vi "InsertMTtemp2DB.vi"(8 "error in (no error)":errorcluster, 9 "Entity":string="QAMT03", 11 "file (use dialog)":path=path "C:/temp/RunTemp/TesterTempByNow.txt") -> (0 "error out":errorcluster)   [LabVIEW 2012]
uses:
  <vilib>/Utility/file.llb/Read From Spreadsheet File (string).vi
  <vilib>/addons/database/Connection.llb/DB Tools Open Connec (Path).vi
  <vilib>/addons/database/Connection.llb/Conn Execute.vi
  <vilib>/addons/database/Recordset.llb/Rec Fetch Integer Data (R).vi
  <vilib>/addons/database/Recordset.llb/Rec Destroy - Connection.vi
  <vilib>/addons/database/NI_Database_API.lvlib
panel:
  in  "Cluster":T1
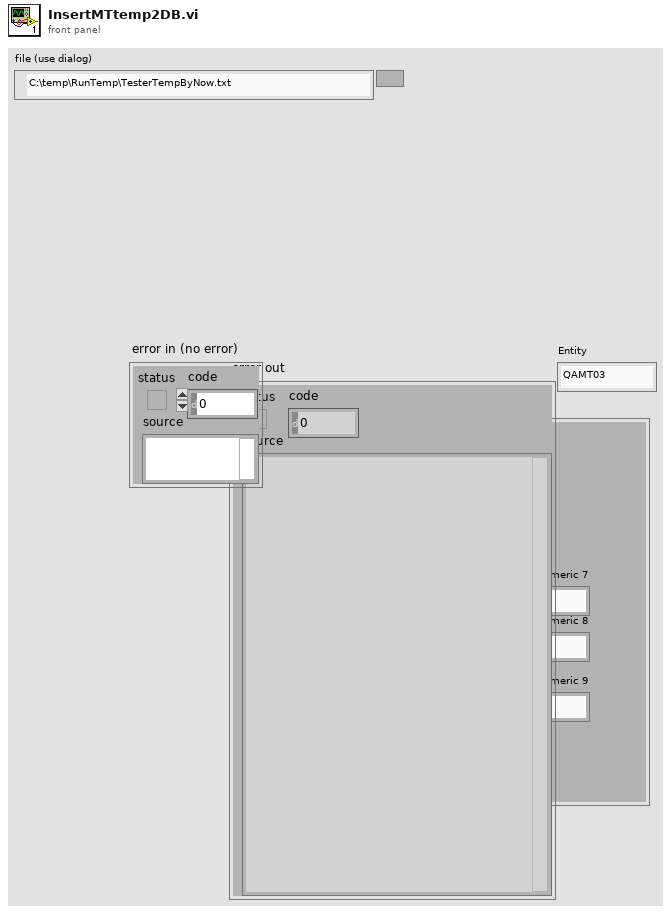
[diagram p1: front panel]
types:
  T1 = cluster{"Entity":string, "Time":string, "Numeric":dbl, "Numeric 2":dbl, "Numeric 3":dbl, "Numeric 4":dbl, "Numeric 5":dbl, "Numeric 6":dbl, "Numeric 7":dbl, "Numeric 8":dbl, "Numeric 9":dbl}
  T2 = typedef "NI_Database_API.lvlib/Conn ObjectReference.ctl" = refnum<k1>
  T3 = typedef "NI_Database_API.lvlib/Rec ObjectReference.ctl" = refnum<k1>
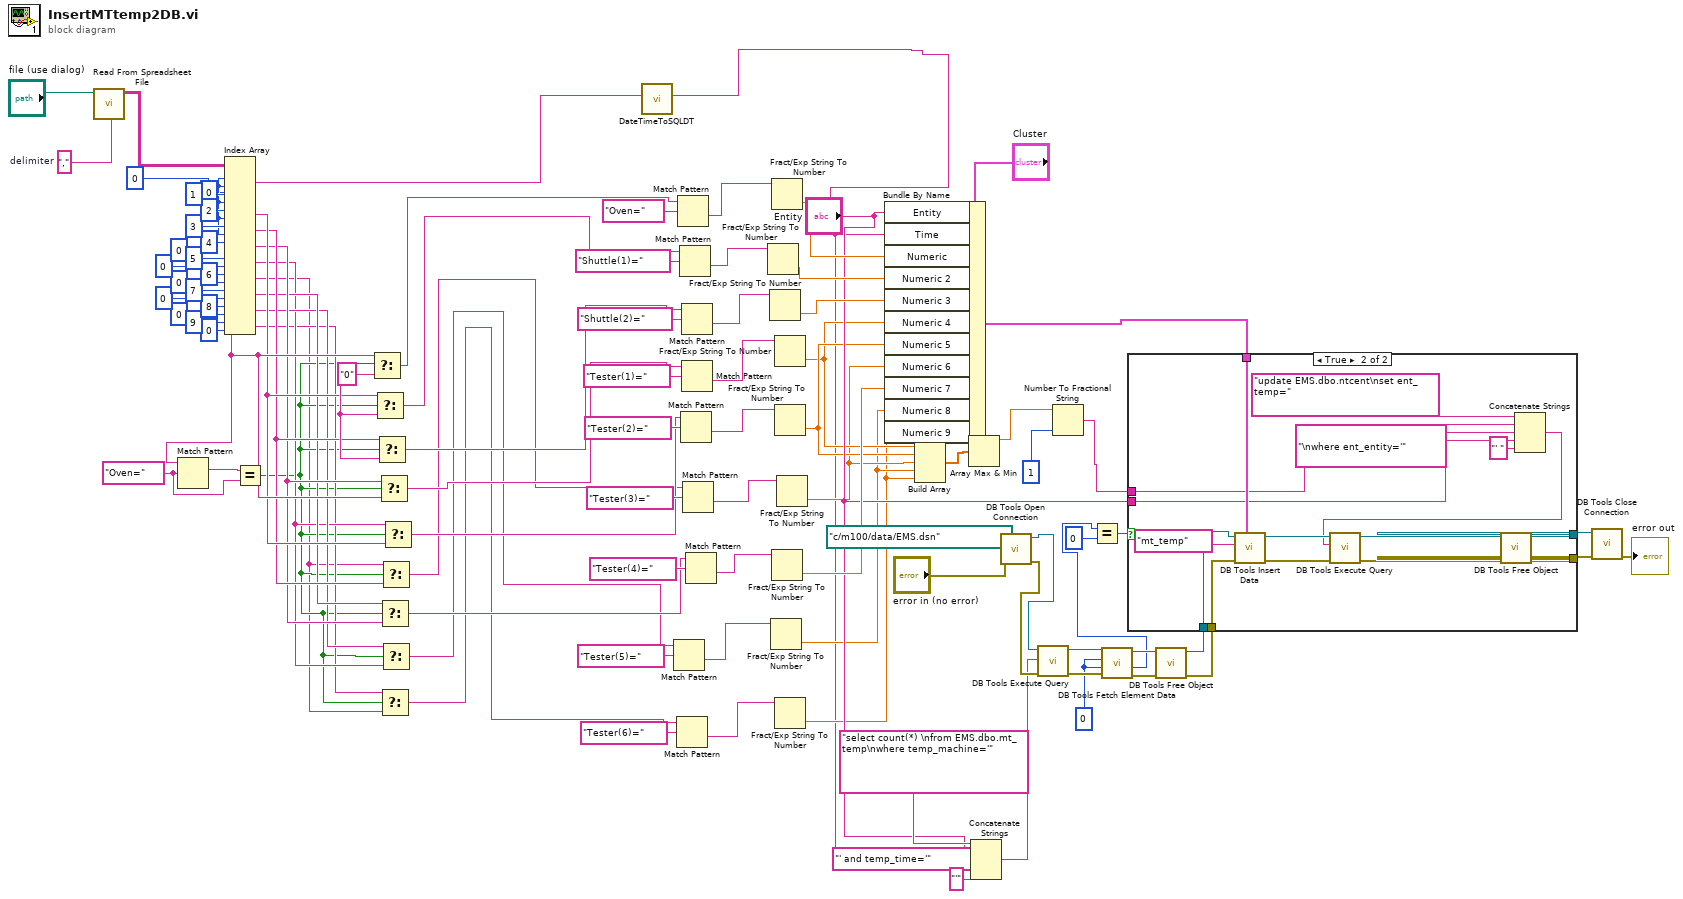
[diagram p0: block diagram]
diagram:
  w29 = "0" ("f")
  w32 = "Oven=" ("regular expression")
  w41 = 0
  (unwired) 0 ("index (col)")
  w86 = 0 ("index (row)")
  w98 = ","  # delimiter
  n1 = call-poly <vilib>:"Read From Spreadsheet File.vi"("delimiter (\\t)"=w98, "file path (dialog if empty)"="file (use dialog)") -> ("all rows"=w61:string[][])  [unwired: 5 in, 4 out]
  n2 = Index Array(array=w61, index (row) #1=w86, index (col) #1=w86, index (row) #2=1 ("index (row)"), index (col) #2=w86, index (row) #3=2 ("index (row)"), index (col) #3=w86, index (row) #4=3 ("index (row)"), index (col) #4=w86, index (row) #5=4 ("index (row)"), index (col) #5=0 ("disabled index (col)"), index (row) #6=5 ("index (row)"), index (col) #6=0 ("disabled index (col)"), index (row) #7=6 ("index (row)"), index (col) #7=0 ("disabled index (col)"), index (row) #8=7 ("index (row)"), index (col) #8=0 ("disabled index (col)"), index (row) #9=8 ("index (row)"), index (col) #9=0 ("disabled index (col)"), index (row) #10=9 ("index (row)"), index (col) #10=0 ("disabled index (col)")) -> (element #1=w2:string, element #2=w27:string, element #3=w25:string, element #4=w22:string, element #5=w21:string, element #6=w16:string, element #7=w12:string, element #8=w20:string, element #9=w18:string, element #10=w15:string)
  n3 = Match Pattern(string=w27, regular expression=w32) -> (match substring=w33:string)  [unwired: 1 in, 3 out]
  n4 = Equal?(x=w33, y=w32) -> (x = y?=w13:bool)
  n5 = Select(t=w27, s=w13, f=w29) -> (s? t:f=w31:string)
  n6 = Select(t=w25, s=w13, f=w29) -> (s? t:f=w30:string)
  n7 = Select(t=w22, s=w13, f=w29) -> (s? t:f=w28:string)
  n8 = Select(t=w21, s=w13, f=w27) -> (s? t:f=w26:string)
  n9 = Select(t=w20, s=w13, f=w21) -> (s? t:f=w19:string)
  n10 = Select(t=w15, s=w13, f=w12) -> (s? t:f=w14:string)
  n11 = Select(t=w12, s=w13, f=w22) -> (s? t:f=w23:string)
  n12 = Select(t=w18, s=w13, f=w16) -> (s? t:f=w17:string)
  n13 = Select(t=w16, s=w13, f=w25) -> (s? t:f=w24:string)
  n14 = call "DateTimeToSQLDT.vi"("DateTimeString"=w2) -> ("SQLDateTime"=w1:string)  [unwired: 10 in]
  n15 = Match Pattern(string=w17, regular expression="Tester(5)=") -> (after substring=w64:string)  [unwired: 1 in, 3 out]
  n16 = Match Pattern(string=w14, regular expression="Tester(6)=") -> (after substring=w63:string)  [unwired: 1 in, 3 out]
  n17 = Match Pattern(string=w31, regular expression="Oven=") -> (after substring=w70:string)  [unwired: 1 in, 3 out]
  n18 = Match Pattern(string=w30, regular expression="Shuttle(1)=") -> (after substring=w71:string)  [unwired: 1 in, 3 out]
  n19 = Match Pattern(string=w24, regular expression="Tester(2)=") -> (after substring=w67:string)  [unwired: 1 in, 3 out]
  n20 = Match Pattern(string=w28, regular expression="Shuttle(2)=") -> (after substring=w69:string)  [unwired: 1 in, 3 out]
  n21 = Match Pattern(string=w26, regular expression="Tester(1)=") -> (after substring=w68:string)  [unwired: 1 in, 3 out]
  n22 = Match Pattern(string=w23, regular expression="Tester(3)=") -> (after substring=w66:string)  [unwired: 1 in, 3 out]
  n23 = Match Pattern(string=w19, regular expression="Tester(4)=") -> (after substring=w65:string)  [unwired: 1 in, 3 out]
  n24 = Fract/Exp String To Number(string=w71) -> (number=w60:dbl)  [unwired: 3 in, 1 out]
  n25 = Fract/Exp String To Number(string=w69) -> (number=w59:dbl)  [unwired: 3 in, 1 out]
  n26 = Fract/Exp String To Number(string=w64) -> (number=w6:dbl)  [unwired: 3 in, 1 out]
  n27 = Fract/Exp String To Number(string=w70) -> (number=w35:dbl)  [unwired: 3 in, 1 out]
  n28 = Fract/Exp String To Number(string=w65) -> (number=w58:dbl)  [unwired: 3 in, 1 out]
  n29 = Fract/Exp String To Number(string=w68) -> (number=w8:dbl)  [unwired: 3 in, 1 out]
  n30 = Fract/Exp String To Number(string=w67) -> (number=w9:dbl)  [unwired: 3 in, 1 out]
  n31 = Fract/Exp String To Number(string=w63) -> (number=w5:dbl)  [unwired: 3 in, 1 out]
  n32 = Fract/Exp String To Number(string=w66) -> (number=w7:dbl)  [unwired: 3 in, 1 out]
  n33 = Bundle By Name(cluster="Cluster", "Entity"="Entity", "Time"=w1, "Numeric"=w35, "Numeric 2"=w60, "Numeric 3"=w59, "Numeric 4"=w8, "Numeric 5"=w9, "Numeric 6"=w7, "Numeric 7"=w58, "Numeric 8"=w6, "Numeric 9"=w5) -> (w53:T1)
  n34 = Build Array(w8, w9, w7, w6, w5) -> (w4:dbl[])
  n35 = Array Max & Min(array=w4) -> (max value=w3:dbl)  [unwired: 3 out]
  n36 = Concatenate Strings("select count(*) \nfrom EMS.dbo.mt_temp\nwhere temp_machine='" ("string"), "Entity", "' and temp_time='" ("string"), w1, "'" ("string")) -> (w36:string)
  n37 = call-poly <vilib>:"DB Tools Open Connection.vi"("error in (no error)"="error in (no error)", "connection information"=path "c:/m100/data/EMS.dsn") -> ("error out"=w46:errorcluster, "connection reference"=w47:T2)  [unwired: 6 in]
  n38 = call-poly <vilib>:"DB Tools Execute Query.vi"("error in (no error)"=w46, "SQL query"=w36, "connection reference"=w47) -> ("error out"=w50:errorcluster, "recordset reference"=w49:T3)  [unwired: 5 in]
  n39 = Number To Fractional String(number=w3, precision (6)=i16 1 ("width (-)")) -> (F-format string=w11:string)  [unwired: 2 in]
  n40 = call-poly <vilib>:"DB Tools Fetch Element Data.vi"("error in (no error)"=w50, "type"=w41, "column index"=w41, "recordset reference"=w49) -> ("error out"=w51:errorcluster, "data"=w42:i32, "recordset reference out"=w48:T3)  [unwired: 3 in]
  n41 = Equal?(x=w42, y=0) -> (x = y?=w43:bool)
  n42 = call-poly <vilib>:"DB Tools Free Object.vi"("error in (no error)"=w51, "recordset reference"=w48) -> ("error out"=w44:errorcluster, "connection reference"=w45:T2)  [unwired: 8 in]
  n43 = case shown="True" w43 {
    tunnel: [w100 w111] -> w56
    tunnel: [w99 w109] -> w55
    tunnel: w53 -> [_ w115]
    tunnel: w45 -> [w100 w114]
    tunnel: w44 -> [w99 w113]
    tunnel: w11 -> [_ w105]
    tunnel: "Entity" -> [_ w103]
    frame False {
    }
    frame True {
      n44 = call <vilib>:"DB Tools Insert Data.vi"("data"=w115, "error in (no error)"=w113, "table"="mt_temp", "connection reference"=w114) -> ("error out"=w110:errorcluster, "connection reference out"=w112:T2)  [unwired: 6 in]
      n45 = Concatenate Strings("update EMS.dbo.ntcent\nset ent_temp=" ("string"), w105, "\nwhere ent_entity='" ("string"), w103, "' " ("string")) -> (w101:string)
      n46 = call-poly <vilib>:"DB Tools Execute Query.vi"("error in (no error)"=w110, "SQL query"=w101, "connection reference"=w112) -> ("error out"=w107:errorcluster, "recordset reference"=w108:T3)  [unwired: 5 in]
      n47 = call-poly <vilib>:"DB Tools Free Object.vi"("error in (no error)"=w107, "recordset reference"=w108) -> ("error out"=w109:errorcluster, "connection reference"=w111:T2)  [unwired: 8 in]
    }
  }
  n48 = call <vilib>:"DB Tools Close Connection.vi"("error in (no error)"=w55, "connection reference"=w56) -> ("error out"=→"error out":errorcluster)  [unwired: 5 in]
